vi "콜라자판기.vi"() -> ()   [LabVIEW 2014]
uses:
  Status.ctl
panel:
  out "그림 링":u16(ring)
  in  "종료":bool
  in  "반환":bool
  in  "구매":bool
  out "투입금액":i32 format="%.0f원"
  in  "동전":T1
  # "콜라자판기"
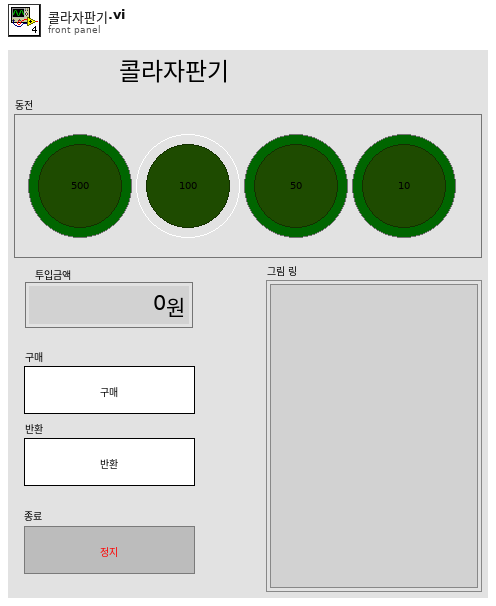
[diagram p1: front panel]
types:
  T1 = cluster{"불리언":bool, "불리언 2":bool, "불리언 3":bool, "불리언 4":bool}
  T2 = typedef "Status.ctl" = enum16{"Idle", "초기화", "종료", "구매", "반환", "1초 기다림"}
  T3 = enum8{"Enabled", "Disabled", "Disabled and Grayed Out"}
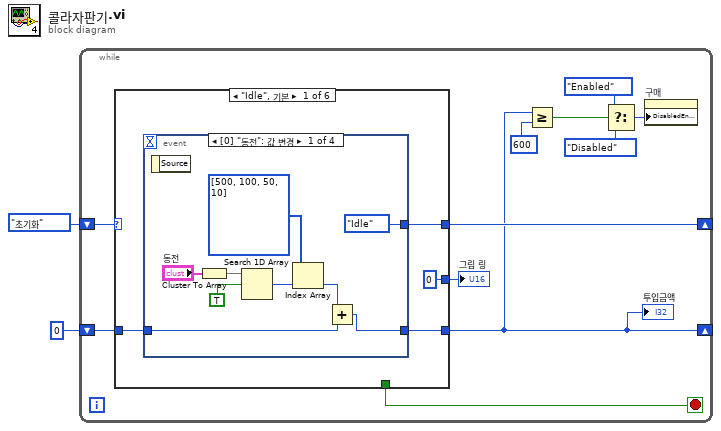
[diagram p0: block diagram]
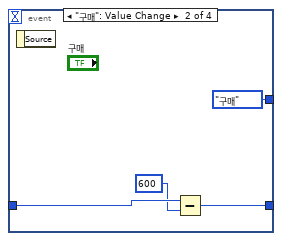
[diagram p2: hidden frame]
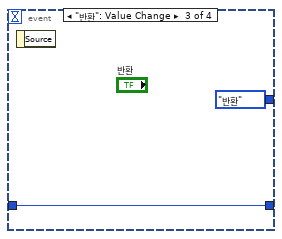
[diagram p3: hidden frame]
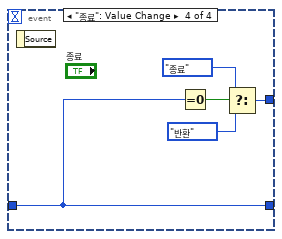
[diagram p4: hidden frame]
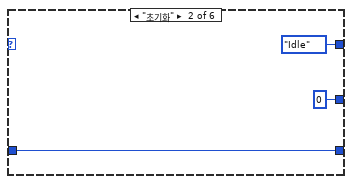
[diagram p5: hidden frame]
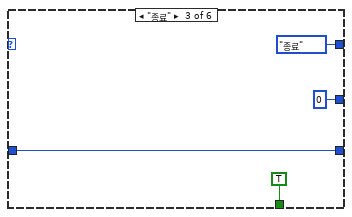
[diagram p6: hidden frame]
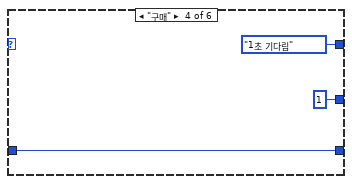
[diagram p7: hidden frame]
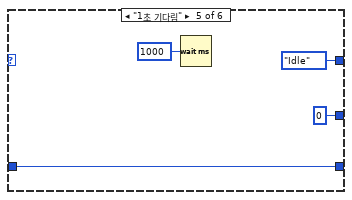
[diagram p8: hidden frame]
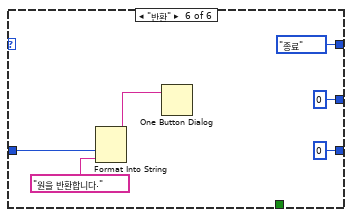
[diagram p9: hidden frame]
diagram:
  n1 = while {
    shift-right: [w12] -> _
    shift-left: Status."초기화" ("Status") -> [w13]
    shift-right: [w4] -> _
    shift-left: 0 -> [w11]
    stop <- w5 stop-if-true
    n2 = case shown="\"Idle\", 기본" w13 {
      tunnel: [w17 Status."Idle" ("Status") Status."종료" ("Status") Status."1초 기다림" ("Status") Status."Idle" ("Status") Status."종료" ("Status")] -> w12
      tunnel: w11 -> [w16 w38 w42 w45 w49 w57]
      tunnel: [w15 w38 w42 w45 w49 0] -> w4
      tunnel: [u16 0 u16 0 u16 0 u16 1 u16 0 u16 0] -> w3
      tunnel: [_ _ TRUE _ _ _] -> w5
      frame "Idle", Default {
        n3 = event shown="[0] \"동전\": 값 변경" {
          selector: _ -> [_ _ _ _]
          dyn-events: _ -> [_ _ _ _]
          timeout: _ -> [_ _ _ _]
          tunnel: [Status."Idle" ("Status") Status."구매" ("Status") Status."반환" ("Status") w33] -> w17
          tunnel: w16 -> [w19 w29 w31 w36]
          tunnel: [w18 w28 w31 w36] -> w15
          event "동전": Value Change {
            n4 = event-data() -> ()  [unwired: 1 in, 1 out]
            n5 = Cluster To Array(cluster="동전") -> (array=w24:bool[])
            n6 = Search 1D Array(1D array=w24, element=TRUE) -> (index of element=w22:i32)  [unwired: 1 in]
            n7 = Index Array(array=i32[] [500, 100, 50, 10], index=w22) -> (element=w20:i32)
            n8 = Add(x=w20, y=w19) -> (x+y=w18:i32)
          }
          event "구매": Value Change {
            n9 = event-data() -> ()  [unwired: 1 in, 1 out]
            n10 = Subtract(x=w29, y=600) -> (x-y=w28:i32)
          }
          event "반환": Value Change {
            n11 = event-data() -> ()  [unwired: 1 in, 1 out]
          }
          event "종료": Value Change {
            n12 = event-data() -> ()  [unwired: 1 in, 1 out]
            n13 = Equal To 0?(x=w36) -> (x = 0?=w37:bool)
            n14 = Select(t=Status."종료" ("Status"), s=w37, f=Status."반환" ("Status")) -> (s? t:f=w33:T2)
          }
        }
      }
      frame "초기화" {
      }
      frame "종료" {
      }
      frame "구매" {
      }
      frame "1초 기다림" {
        n15 = Wait (ms)(milliseconds to wait=u32 1000 ("대기 시간(ms)")) -> ()  [unwired: 1 out]
      }
      frame "반환" {
        n16 = Format Into String(w57, "원을 반환합니다.") -> (resulting string=w55:string)  [unwired: 3 in, 1 out]
        n17 = One Button Dialog(message=w55) -> ()  [unwired: 1 in, 1 out]
      }
    }
    "투입금액" <- w4
    "그림 링" <- w3
    n18 = Greater Or Equal?(x=w4, y=600) -> (x >= y?=w9:bool)
    n19 = Select(t=T3."Enabled" ("비활성화"), s=w9, f=T3."Disabled" ("비활성화")) -> (s? t:f=w6:T3)
    n20 = property on="구매" class="Bool"("DisabledEnum"=w6) -> ()  [unwired: 2 in, 2 out]
  }
